vi "TEST_bench_FXP_ss_matmult.vi"() -> ()   [LabVIEW 2017]
uses:
  <vilib>/Platform/TimedLoop/XDataNode/timing_clust.ctl
  <vilib>/Platform/TimedLoop/XDataNode/nitl_modes.ctl
  <vilib>/Platform/TimedLoop/XDataNode/wakeup.ctl
  fpga_subVIs_ssxy/fixed-point-ss/typeDefs/x_vec_bram.ctl
  fpga_subVIs_ssxy/fixed-point-ss/typeDefs/A_as_vec_bram.ctl
  <vilib>/rvi/Emulation/niFpgaSctlEmulationGetInTimedLoop.vi
  <vilib>/rvi/Emulation/niFpgaEmulationReportErrorSimple.vi
  <vilib>/rvi/Emulation/niFpgaGetClockAttributes.vi
  <vilib>/rvi/Emulation/niFpgaCriticalErrorInLSC.vi
  <vilib>/rvi/DataTransferAndStorage/Container/Common/niFpgaContainerExecOnDevCompGetState.vi
  <vilib>/rvi/Emulation/niFpgaEmulationIsFPGAContextNoSignature.vi
  <vilib>/rvi/DataTransferAndStorage/Container/Common/niFpgaContainerGetUniqueNameForEmu.vi
  <vilib>/rvi/Emulation/niFpgaProcessEmulError.vi
  <vilib>/rvi/errors/nirviReportUnexpectedCaseInternalError (U32).vi
  <vilib>/rvi/Memory/Memory_Emulation/niFpgaMemoryEmulationCacheClearOnFirstRun.vi
  <vilib>/rvi/Memory/Memory_Emulation/nirvimemoryEmulationManagerCache_MakeExclusive.vi
  <vilib>/rvi/Memory/Memory_Emulation/niFpgaMemoryEmulationValidateCache.vi
  <vilib>/rvi/Memory/Memory_Emulation/nirvimemoryEmulationManagerCache_InsertValue.vi
  <vilib>/Utility/error.llb/Clear Errors.vi
  <vilib>/rvi/Memory/Memory_Emulation/nirvimemoryEmulationManagerCache_ReleaseExclusive.vi
  <vilib>/rvi/Memory/Memory_Emulation/nirvimemoryEmulationManagerCache_GetValue.vi
  <vilib>/rvi/Memory/Memory_Emulation/nirvimemoryEmulationManagerCache_SetValue.vi
  <vilib>/rvi/Emulation/niFpgaSctlEmulationResourceMgr.vi
  <vilib>/Platform/TimedLoop/XDataNode/XDataNode.xnode
  <vilib>/rvi/DataTransferAndStorage/Container/XNode/niFpgaContainer.xnode
  <vilib>/rvi/Memory/Memory_Emulation/niFpgaMemoryEmulationRefIn.vi
  <vilib>/Platform/TimedLoop/XDataNode/XDNodeRunTimeDep.lvlib
panel:
  out "xk_01":fxp<+/-,32,6>[](array[numeric])
  out "xk_10":fxp<+/-,32,6>[](array[numeric])
  out "Uk 2":fxp<+/-,32,6>
  out "Numeric":i32
  out "Yk":fxp<+/-,36,13>[](array[numeric])
  in  "Uk":fxp<+/-,32,6>[](array[numeric])
  in  "ABCD_col":fxp<+/-,32,6>[](array[numeric])
  in  "Ns_nsw":u8=9
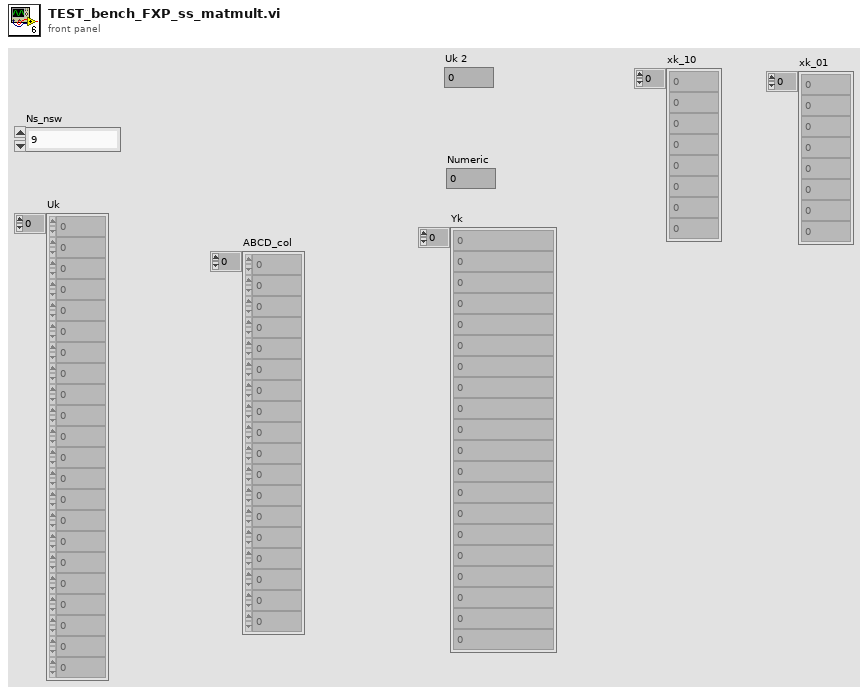
[diagram p1: front panel]
types:
  T1 = typedef "x_vec_bram.ctl" = refnum<k21>
  T2 = typedef "XDNodeRunTimeDep.lvlib/timing_clust.ctl" = cluster{"Expected End [f-1]":u64, "Actual End [f-1]":u64, "Finished Late? [f-1]":bool, "Expected End [i-1]":u64, "Actual End [i-1]":u64, "Finished Late? [i-1]":bool, "Expected Start [i]":u64, "Actual Start [i]":u64, "Expected Start [f]":u64, "Actual Start [f]":u64, "Source Name":string, "Structure Name":string, "Period":i64, "Deadline":i64, "Offset":i64, "Start":i64, "Priority":i32, "Timeout":i32, "Mode":T3, "Wakeup Reason":T4, "Error":errorcluster, "Source Type":string, "Secondary Source Type":string, "Global End Time":u64, "Global Start Time":u64, "Frame Duration":u64, "Iteration Duration":u64, "Assigned CPU":i32, "I/O Scan Engine Mode":u32}
  T3 = typedef "XDNodeRunTimeDep.lvlib/nitl_modes.ctl" = enum32{"No Change", "Process missed periods, maintain original phase", "Discard missed periods, maintain original phase", "Process missed periods, ignore original phase", "Discard missed periods, ignore original phase"}
  T4 = typedef "XDNodeRunTimeDep.lvlib/wakeup.ctl" = enum32{"Normal", "Aborted", "Asynchronous wakeup", "Timing source error", "Timed loop error", "Timeout"}
  T5 = typedef "A_as_vec_bram.ctl" = refnum<k21>
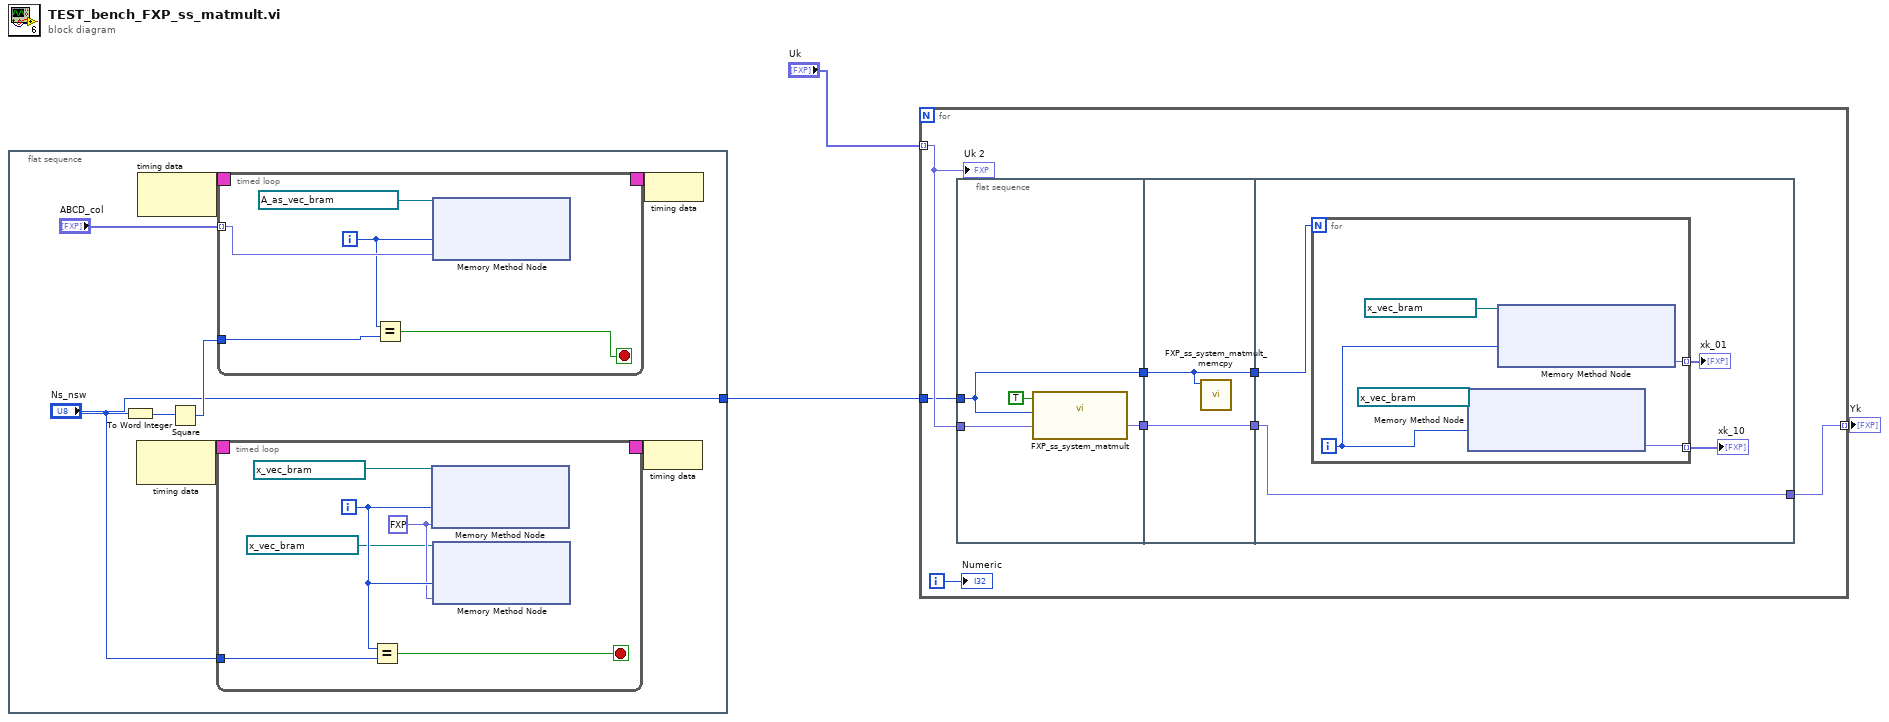
[diagram p0: block diagram]
diagram:
  n1 = flat-sequence {
    tunnel: ["Ns_nsw"] -> w1
    frame #0 {
      n2 = To Word Integer(number="Ns_nsw") -> (16bit integer=w6:i16)
      n3 = node-c288() -> (w9:T2)  [unwired: 1 in]
      n4 = node-c288() -> (w11:T2)  [unwired: 1 in]
      n5 = Square(x=w6) -> (x^2=w5:i16)
      n6 = timed-loop {
        timing: w9 -> [_]
        timing-out: [_] -> w8
        tunnel: "Ns_nsw" -> [w15]
        i -> [w14]
        stop <- w17 stop-if-true
        w13 = fxp<+/-,32,6> 0.0 ("Uk")
        n7 = Equal?(x=w14, y=w15) -> (x = y?=w17:bool)
        n8 = xnode ("Memory Method Node")("Address"=w14, "Data"=w13, "Memory In"=T1 "xk_0_1_zaxis" ("Memory")) -> ()  [unwired: 1 out]
        n9 = xnode ("Memory Method Node")("Address"=w14, "Data"=w13, "Memory In"=T1 "xk_1_0_zaxis" ("Memory")) -> ()  [unwired: 1 out]
      }
      n10 = timed-loop {
        timing: w11 -> [_]
        timing-out: [_] -> w10
        tunnel: "ABCD_col" -> [w25] mode=indexing
        tunnel: w5 -> [w22]
        i -> [w23]
        stop <- w24 stop-if-true
        n11 = Equal?(x=w23, y=w22) -> (x = y?=w24:bool)
        n12 = xnode ("Memory Method Node")("Address"=w23, "Data"=w25, "Memory In"=T5 "AasCol_FXP_zaxis") -> ()  [unwired: 1 out]
      }
      n13 = node-c288(w8) -> ()
      n14 = node-c288(w10) -> ()
    }
  }
  n15 = for {
    tunnel: w1 -> [w37]
    tunnel: "Uk" -> [w38] mode=indexing
    tunnel: [w31] -> w2 mode=indexing
    i -> [w34]
    n16 = flat-sequence {
      tunnel: w38 -> [w42]
      tunnel: w37 -> [w40]
      tunnel: [w41] -> w36
      tunnel: [w40] -> w35
      tunnel: w36 -> [w44]
      tunnel: w35 -> [w43]
      tunnel: [w44] -> w33
      tunnel: [w43] -> w32
      tunnel: w33 -> [w48]
      tunnel: [w48] -> w31
      tunnel: w32 -> [w46]
      frame #0 {
        n17 = call "FXP_ss_system_matmult.vi"("Uk"=w42, "Ns_nsw"=w40, "inputValid"=TRUE) -> ("Yk"=w41:fxp<+/-,36,13>)  [unwired: 7 in, 1 out]
      }
      frame #1 {
        n18 = call "FXP_ss_system_matmult_memcpy.vi"("Ns_nsw"=w43) -> ()  [unwired: 11 in]
      }
      frame #2 {
        n19 = for {
          N: w46 -> [_]
          tunnel: [w52] -> w47 mode=indexing
          tunnel: [w49] -> w45 mode=indexing
          i -> [w50]
          n20 = xnode ("Memory Method Node")("Address"=w50, "Memory In"=T1 "xk_1_0_zaxis" ("Memory")) -> ("Data"=w52:fxp<+/-,32,6>)  [unwired: 1 out]
          n21 = xnode ("Memory Method Node")("Address"=w50, "Memory In"=T1 "xk_0_1_zaxis" ("Memory")) -> ("Data"=w49:fxp<+/-,32,6>)  [unwired: 1 out]
        }
        "xk_10" <- w47
        "xk_01" <- w45
      }
    }
    "Numeric" <- w34
    "Uk 2" <- w38
  }
  "Yk" <- w2
